vi "DrivePID.vi"(7 "Compensate":bool, 9 "SetpointRight":dbl format="%.2f", 11 "SetpointLeft":dbl format="%.2f") -> (15 "Done":bool)   [LabVIEW 2014]
uses:
  <vilib>/Rock Robotics/WPI/RobotDrive/WPI_RobotDriveGetSetRefNum.vi
  Robot Global Data.vi
  <vilib>/addons/control/pid/pid.llb/PID (DBL).vi
  <vilib>/addons/control/pid/NI_PID_pid.lvlib
panel:
  out "Right Graph":dbl[](graph)
  out "Left Graph":dbl[](graph)
  out "Timing":dbl
  in  "PID gains for motor gain":T1={"proportional gain (Kc)"=1.0, "integral time (Ti, min)"=0.01, "derivative time (Td, min)"=0.0} {"derivative time (Td, min)" format="%.3f"; "integral time (Ti, min)" format="%.3f"; "proportional gain (Kc)" format="%.3f"}
  in  "LeftDriveRefNum":string="My Encoder RefNum"
  in  "RightDriveRefNum":string="My Encoder RefNum"
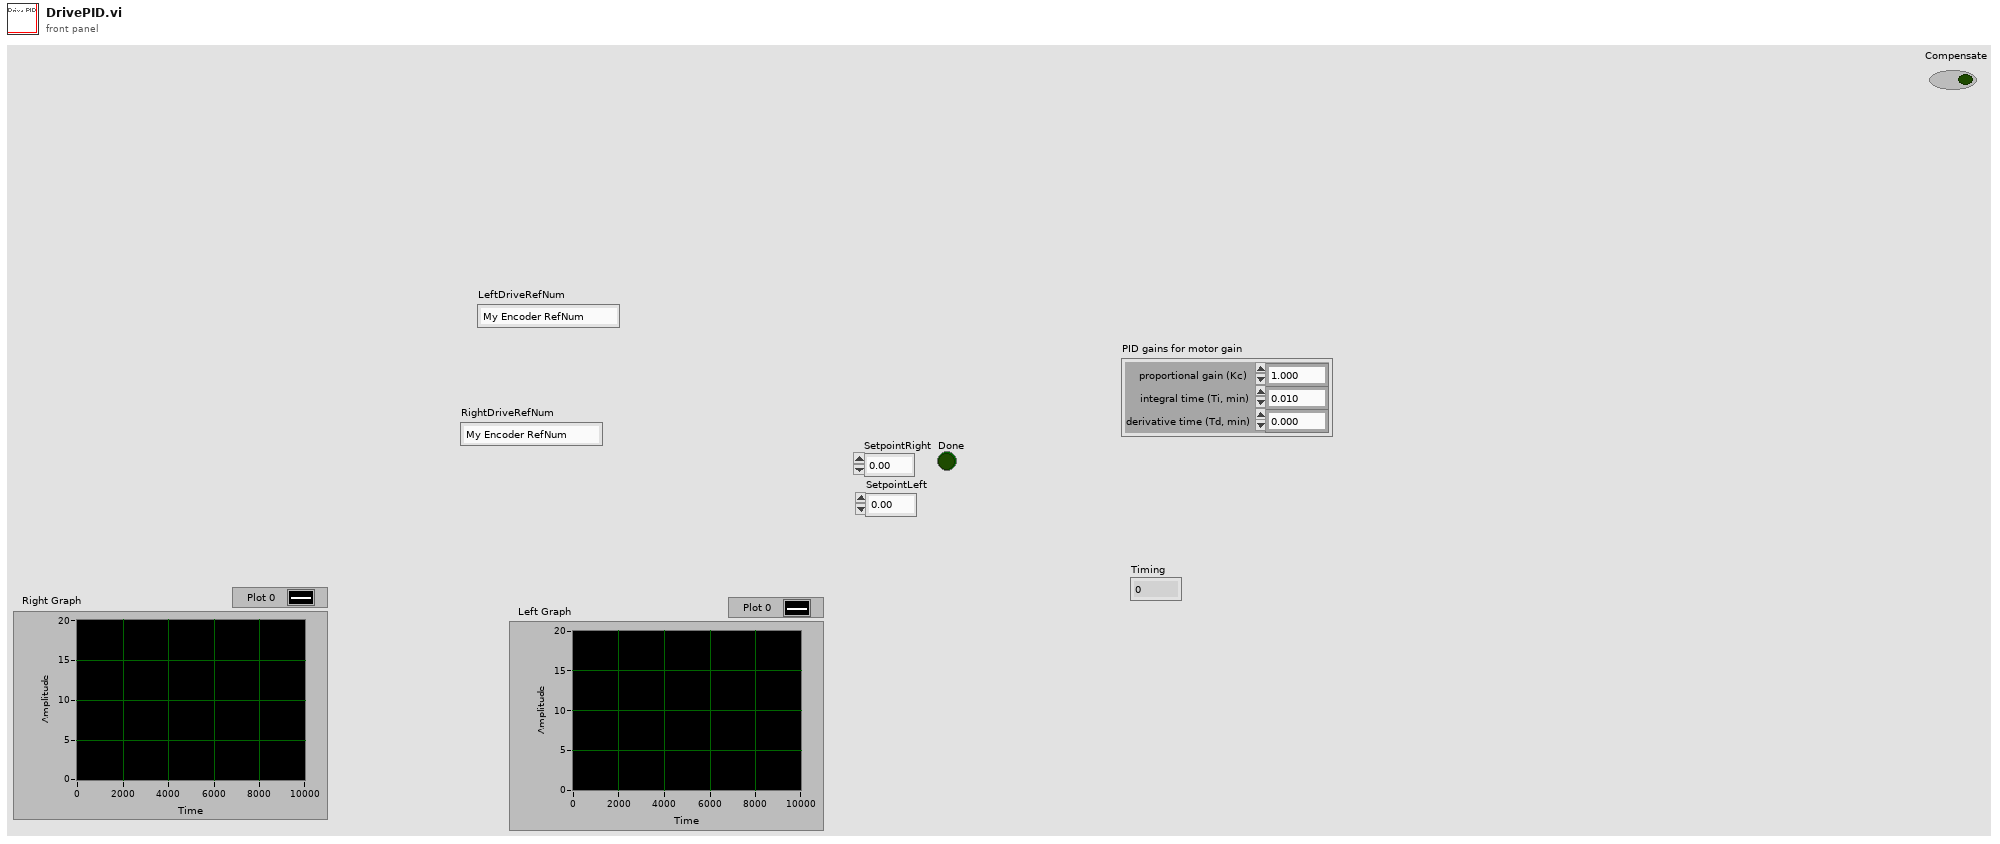
[diagram p1: front panel]
types:
  T1 = cluster{"proportional gain (Kc)":dbl, "integral time (Ti, min)":dbl, "derivative time (Td, min)":dbl}
  T2 = typedef "WPI_EncoderDevRef.ctl" = cluster{"DevStatus":errorcluster, "EncoderIndex":T3, "CounterIndex":T4, "DistancePerCount":dbl, "Decoding Type":T5}
  T3 = typedef "FPGA_EncoderIdx.ctl" = enum8{"Enc 0", "Enc 1", "Enc 2", "Enc 3", "Enc 4", "Enc 5", "Enc 6", "Enc 7", "Invalid"}
  T4 = typedef "FPGA_CounterCtrSystemIndex.ctl" = enum8{"Ctr 0", "Ctr 1", "Ctr 2", "Ctr 3", "Ctr 4", "Ctr 5", "Ctr 6", "Ctr 7", "Invalid"}
  T5 = typedef "WPI_EncoderType.ctl" = enum16{"1x", "2x", "4x"}
  T6 = typedef "WPI_RobotDriveDevRef.ctl" = cluster{"DevStatus":errorcluster, "Motors[]":T7[], "Square Inputs":bool, "Max Output":dbl}
  T7 = typedef "WPI_MotorControlDeviceRef.ctl" = cluster{"DeviceStatus":errorcluster, "Type":T8, "PWM":cluster{"Controller":T9, "PWM Channel":T10, "DeadBand":T11}, "CAN":cluster{"Device Number":u8, "Control Mode":T12, "Semaphore":T13, "Max Vout":dbl, "TalonSRX Control Mode":T14}, "Invert":bool, "TransformRef":T15, "InvTransformRef":T15}
  T8 = typedef "WPI_MotorControlType.ctl" = enum16{"PWM", "CAN", "CANTalonSRX"}
  T9 = typedef "FPGA_TypedefDigitalModule.ctl" = enum16{"Controller 1"}
  T10 = typedef "FPGA_DIOPWMChannel.ctl" = enum8{"PWM 0", "PWM 1", "PWM 2", "PWM 3", "PWM 4", "PWM 5", "PWM 6", "PWM 7", "PWM 8", "PWM 9", "PWM MXP 0", "PWM MXP 1", "PWM MXP 2", "PWM MXP 3", "PWM MXP 4", "PWM MXP 5", "PWM MXP 6", "PWM MXP 7", "PWM MXP 8", "PWM MXP 9", "Invalid"}
  T11 = typedef "WPI_PWMDeadband.ctl" = cluster{"Name":string, "maxPositivePwm":i32, "minPositivePwm":i32, "centerPwm":i32, "maxNegativePwm":i32, "minNegativePwm":i32, "angularRange":u16}
  T12 = typedef "WPI_CANJaguar_ControlMode.ctl" = enum8{"Percent VBus", "Current", "Speed", "Position", "Voltage"}
  T13 = typedef "Semaphore RefNum" = refnum<k1>
  T14 = typedef "WPI_CANTalonSRX_APIControlMode.ctl" = enum8{"Percent VBus", "Speed", "Position", "Slave", "Unchanged / Invalid"}
  T15 = typedef "WPI_PWMTransform_ConPane.ctl" = refnum<vi>
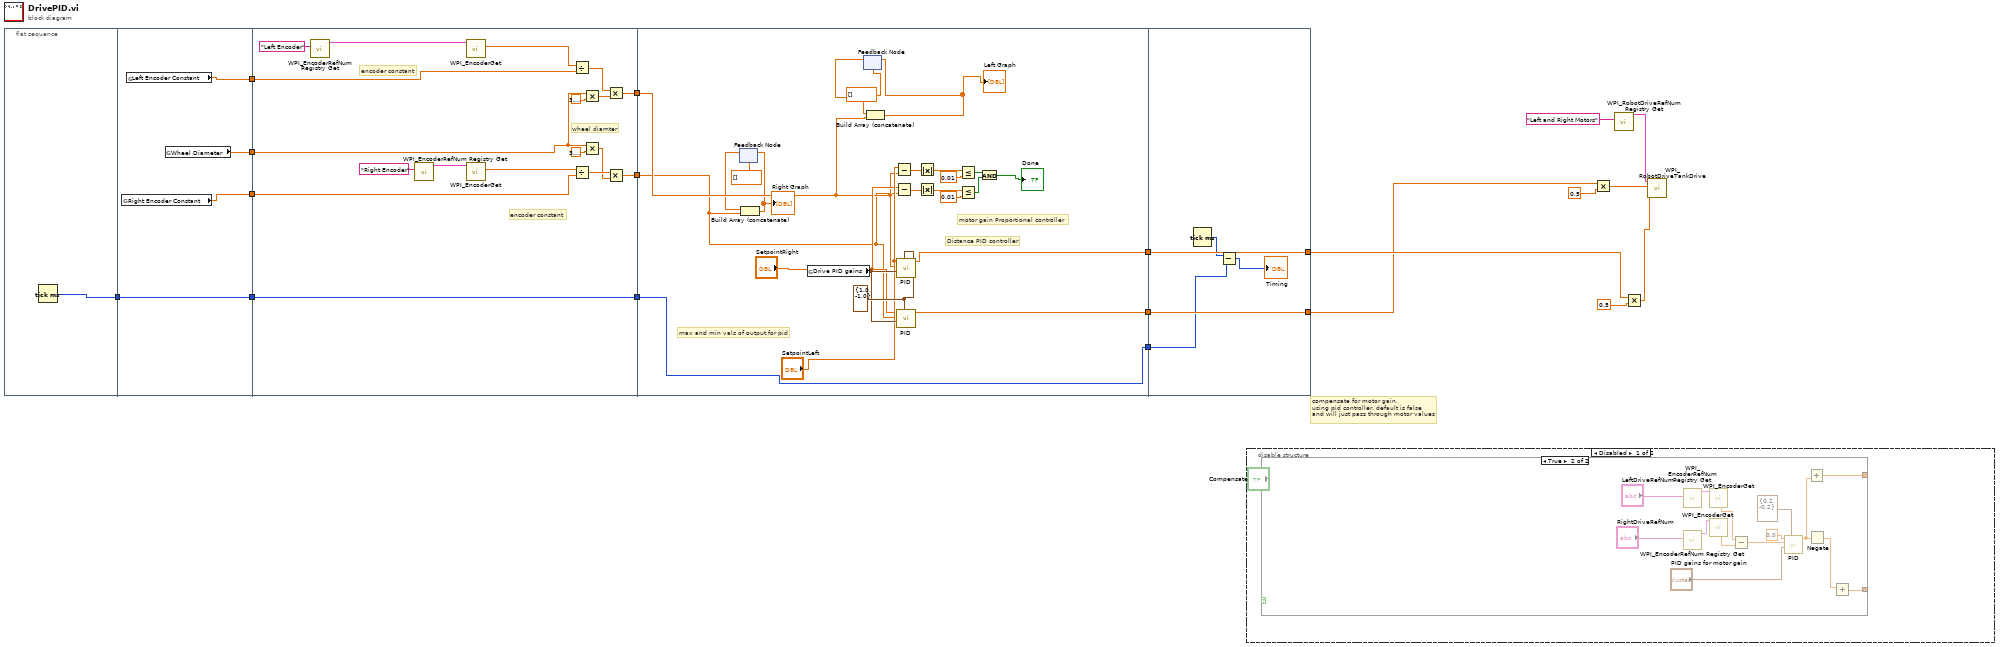
[diagram p0: block diagram]
diagram:
  # "compensate for motor gain,\nusing pid controller. default is false\nand will just pass through motor values"
  n1 = flat-sequence {
    tunnel: [w20] -> w2
    tunnel: [w24] -> w9
    tunnel: [w23] -> w8
    tunnel: [w22] -> w7
    tunnel: [w21] -> w3
    tunnel: w2 -> [w21]
    tunnel: [w34] -> w13
    tunnel: [w31] -> w12
    tunnel: w9 -> [w28]
    tunnel: w8 -> [w27]
    tunnel: w7 -> [w26]
    tunnel: [w25] -> w4
    tunnel: w3 -> [w25]
    tunnel: w13 -> [w50]
    tunnel: w12 -> [w47]
    tunnel: [w56] -> w6
    tunnel: [w55] -> w5
    tunnel: w4 -> [w51]
    tunnel: [w51] -> w1
    tunnel: [w70] -> w10
    tunnel: [w71] -> w11
    tunnel: w6 -> [w71]
    tunnel: w5 -> [w70]
    tunnel: w1 -> [w67]
    frame #0 {
      n2 = Tick Count (ms)() -> (millisecond timer value=w20:u32)
    }
    frame #1 {
      n3 = global read "Robot Global Data.vi" "Right Encoder Constant"() -> (w22:dbl)
      n4 = global read "Robot Global Data.vi" "Left Encoder Constant"() -> (w24:dbl)
      n5 = global read "Robot Global Data.vi" "Wheel Diameter"() -> (w23:dbl)
    }
    frame #2 {
      # "encoder constant"
      # "encoder constant"
      # "wheel diamter"
      n6 = call <vilib>:"WPI_EncoderRefNum Registry Get.vi"("refnum name"="Left Encoder") -> ("EncoderDevRef"=w42:T2)  [unwired: 9 in, 1 out]
      n7 = call <vilib>:"WPI_EncoderRefNum Registry Get.vi"("refnum name"="Right Encoder") -> ("EncoderDevRef"=w41:T2)  [unwired: 9 in, 1 out]
      n8 = call <vilib>:"WPI_EncoderGet.vi"("EncoderDevRef"=w42) -> ("Distance"=w38:dbl)  [unwired: 5 in, 5 out]
      n9 = call <vilib>:"WPI_EncoderGet.vi"("EncoderDevRef"=w41) -> ("Distance"=w37:dbl)  [unwired: 5 in, 5 out]
      n10 = Divide(x=w38, y=w28) -> (x/y=w36:dbl)
      n11 = Divide(x=w37, y=w26) -> (x/y=w33:dbl)
      n12 = Multiply(x=w27, y=3.141592653589793) -> (x*y=w35:dbl)
      n13 = Multiply(x=w27, y=3.141592653589793) -> (x*y=w32:dbl)
      n14 = Multiply(x=w36, y=w35) -> (x*y=w34:dbl)
      n15 = Multiply(x=w33, y=w32) -> (x*y=w31:dbl)
    }
    frame #3 {
      w65 = cluster{"output high":dbl, "output low":dbl} {"output high"=1.0, "output low"=-1.0} ("output range")
      # "max and min vals of output for pid"
      # "motor gain Proportional controller"
      # "Distance PID controller"
      n16 = feedback #1(dbl[] []) -> (w48:dbl[])
      n17 = Build Array (concatenate)(w48, w47) -> (w49:dbl[])
      "Right Graph" <- w49
      n18 = feedback-in #1(w49) -> ()
      n19 = global read "Robot Global Data.vi" "Drive PID gains"() -> (w57:T1)
      n20 = feedback #2(dbl[] []) -> (w43:dbl[])
      n21 = Build Array (concatenate)(w43, w50) -> (w44:dbl[])
      "Left Graph" <- w44
      n22 = feedback-in #2(w44) -> ()
      n23 = Subtract(x="SetpointLeft", y=w50) -> (x-y=w64:dbl)
      n24 = Subtract(x="SetpointRight", y=w47) -> (x-y=w60:dbl)
      n25 = call-poly <vilib>:"PID.vi"("output range"=w65, "PID gains"=w57, "process variable"=w50, "setpoint"="SetpointLeft") -> ("output"=w56:dbl)  [unwired: 6 in, 1 out]
      n26 = call-poly <vilib>:"PID.vi"("output range"=w65, "PID gains"=w57, "process variable"=w47, "setpoint"="SetpointRight") -> ("output"=w55:dbl)  [unwired: 6 in, 1 out]
      n27 = Absolute Value(x=w64) -> (abs(x)=w59:dbl)
      n28 = Absolute Value(x=w60) -> (abs(x)=w58:dbl)
      n29 = Less Or Equal?(x=w59, y=0.01) -> (x <= y?=w61:bool)
      n30 = Less Or Equal?(x=w58, y=0.01) -> (x <= y?=w62:bool)
      n31 = And(x=w61, y=w62) -> (x .and. y?=→"Done":bool)
    }
    frame #4 {
      n32 = Tick Count (ms)() -> (millisecond timer value=w69:u32)
      n33 = Subtract(x=w69, y=w67) -> (x-y=→"Timing":u32)
    }
  }
  n34 = disable-structure shown="Disabled" {
    frame Disabled {
      n35 = case shown="True" {
        selector: _ -> [_ _]
        tunnel: [_ w74] -> _
        tunnel: [_ w72] -> _
        frame False {
        }
        frame True {
          n36 = call <vilib>:"WPI_EncoderRefNum Registry Get.vi"("refnum name"="LeftDriveRefNum") -> ("EncoderDevRef"=w84:T2)  [unwired: 9 in, 1 out]
          n37 = call <vilib>:"WPI_EncoderRefNum Registry Get.vi"("refnum name"="RightDriveRefNum") -> ("EncoderDevRef"=w81:T2)  [unwired: 9 in, 1 out]
          n38 = call <vilib>:"WPI_EncoderGet.vi"("EncoderDevRef"=w84) -> ("Rate"=w79:dbl)  [unwired: 5 in, 5 out]
          n39 = call <vilib>:"WPI_EncoderGet.vi"("EncoderDevRef"=w81) -> ("Rate"=w78:dbl)  [unwired: 5 in, 5 out]
          n40 = Subtract(x=w79, y=w78) -> (x-y=w76:dbl)
          n41 = call-poly <vilib>:"PID.vi"("output range"=cluster{"output high":dbl, "output low":dbl} {"output high"=0.2, "output low"=-0.2}, "PID gains"="PID gains for motor gain", "process variable"=w76, "setpoint"=0.0) -> ("output"=w73:dbl)  [unwired: 6 in, 1 out]
          n42 = Add(y=w73) -> (x+y=w72:dbl)  [unwired: 1 in]
          n43 = Negate(x=w73) -> (-x=w75:dbl)
          n44 = Add(x=w75) -> (x+y=w74:dbl)  [unwired: 1 in]
        }
      }
    }
    frame Enabled {
    }
  }
  n45 = Multiply(x=w10, y=0.5) -> (x*y=w15:dbl)
  n46 = call <vilib>:"WPI_RobotDriveRefNum Registry Get.vi"("refnum name"="Left and Right Motors") -> ("RobotDriveDevRef"=w18:T6)  [unwired: 9 in, 1 out]
  n47 = Multiply(x=w11, y=0.5) -> (x*y=w14:dbl)
  n48 = call <vilib>:"WPI_RobotDriveTankDrive.vi"("Right axis value"=w14, "Left axis value"=w15, "RobotDriveDevRef"=w18) -> ()  [unwired: 6 in, 3 out]
